vi "Get Plot at Mouse Click in Plot Area [AAC].vi"(8 "error in (no error)":errorcluster, 10 "Mouse Click Coordinates (defaut: last plot)":T2={"Horizontal"=2147483647, "Vertical"=0}, 11 "XYGraph Ref":T1) -> (0 "error out":errorcluster, 1 "Plot Index":i32, 3 "XYGraph Ref":T1)   [LabVIEW 2019]
doc: "If the Mouse Coordinates X value = 2147483647 (max I32 value), this means that the last plot is sought for is thus the plot returned.\nIf there is no plot in the Graph, -1 is returned"
uses:
  XY Graph/XY Graph Refnum.ctl
  <vilib>/Utility/miscctls.llb/LVPoint32TypeDef.ctl
  XY Graph/XY Graph Add-Ons.lvlib
panel:
  in  "Array of Array Cluster":cluster{"Array":dbl[], "Array":dbl[]}[](array[cluster])
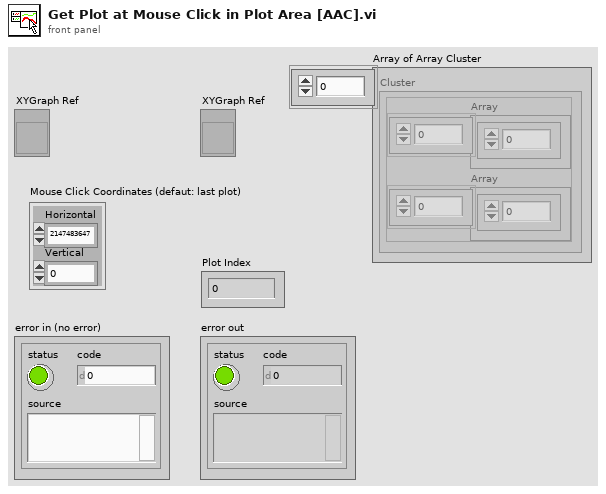
[diagram p1: front panel]
types:
  T1 = typedef "XY Graph Add-Ons.lvlib/XY Graph Refnum.ctl" = refnum<vi>
  T2 = typedef "LVPoint32TypeDef.ctl" = cluster{"Horizontal":i32, "Vertical":i32}
  T3 = typedef "LVRectTypeDef.ctl" = cluster{"Left":i16, "Top":i16, "Right":i16, "Bottom":i16}
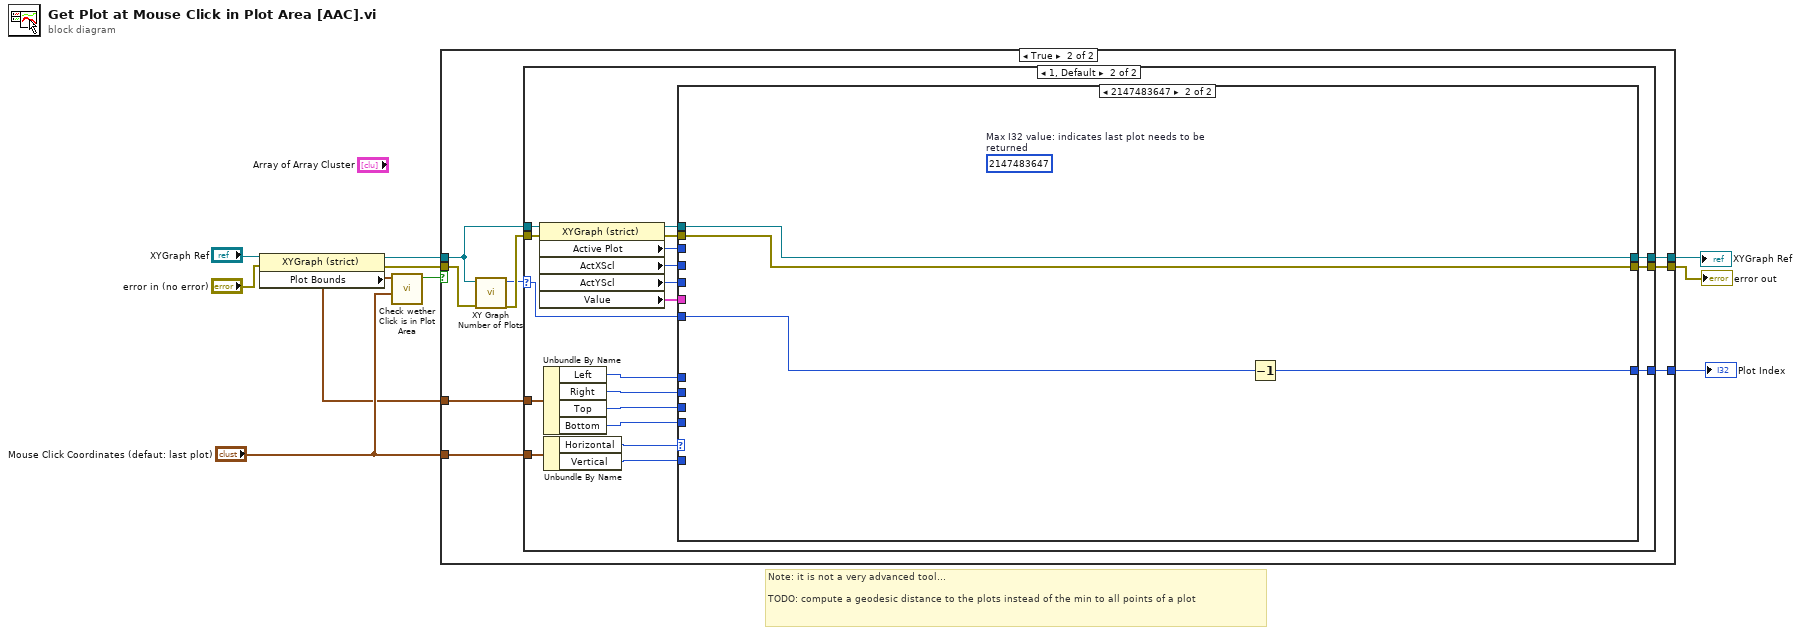
[diagram p0: block diagram]
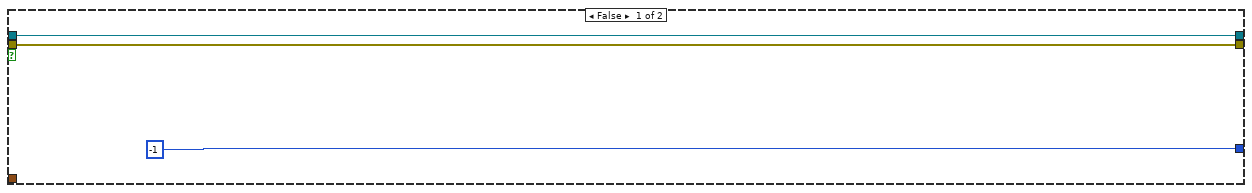
[diagram p2: hidden frame]
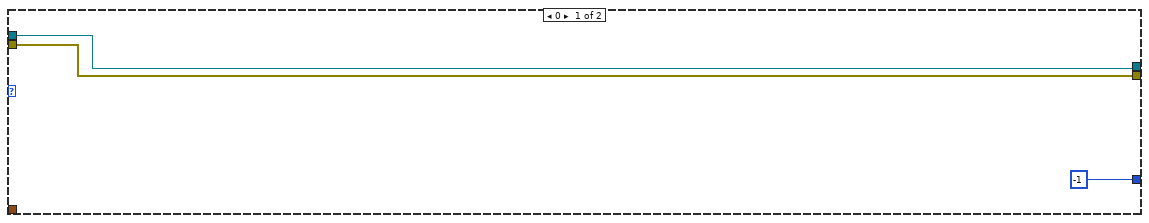
[diagram p3: hidden frame]
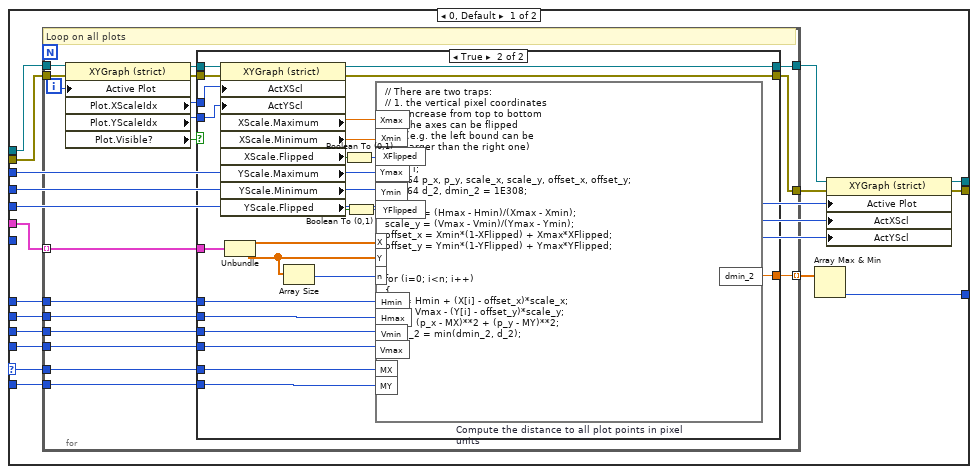
[diagram p4: hidden frame]
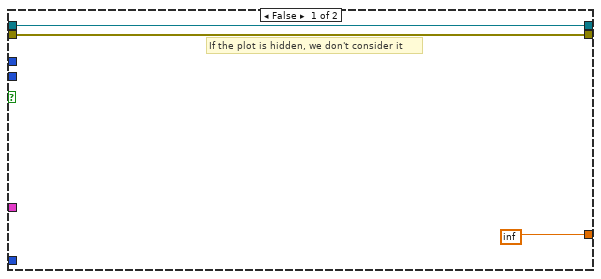
[diagram p5: hidden frame]
diagram:
  # "Note: it is not a very advanced tool...\n\nTODO: compute a geodesic distance to the plots instead of the min to all points of a plot"
  n1 = property class="XYGraph (strict)"(reference="XYGraph Ref", error in="error in (no error)") -> (reference out=w6:T1, error out=w7:errorcluster, "Plot Bounds"=w1:T3)
  n2 = call "Check wether Click is in Plot Area.vi"("Mouse Click Coordinates"="Mouse Click Coordinates (defaut: last plot)", "Plot Bounds"=w1) -> ("Is in Plot Area?"=w8:bool)  [unwired: 9 in]
  n3 = case shown="True" w8 {
    tunnel: w7 -> [w12 w16]
    tunnel: w6 -> [w13 w17]
    tunnel: [w13 w22] -> w5
    tunnel: [w12 w21] -> w4
    tunnel: [-1 ("Plot Index") w18] -> w3
    tunnel: "Mouse Click Coordinates (defaut: last plot)" -> [_ w20]
    tunnel: w1 -> [_ w19]
    frame False {
    }
    frame True {
      n4 = call "XY Graph Number of Plots.vi"("Error In"=w16, "XYGraph in"=w17) -> ("Error Out"=w15:errorcluster, "# Plots"=w14:i32)  [unwired: 8 in]
      n5 = case shown="1, Default" w14 {
        selector: w14 -> [_ w26]
        tunnel: [w24 w45] -> w22
        tunnel: [w23 w44] -> w21
        tunnel: w20 -> [_ w43]
        tunnel: w19 -> [_ w42]
        tunnel: [-1 w41] -> w18
        tunnel: w17 -> [w24 w29]
        tunnel: w15 -> [w23 w28]
        frame 0 {
        }
        frame 1, Default {
          n6 = property class="XYGraph (strict)"(reference=w29, error in=w28) -> (reference out=w40:T1, error out=w27:errorcluster, "Active Plot"=w39:u32, "ActXScl"=w38:i32, "ActYScl"=w37:i32, "Value"=w30:cluster{"X Array":dbl[], "Y Array":dbl[]}[])
          n7 = Unbundle By Name(w42) -> ("Left"=w36:i16, "Right"=w35:i16, "Top"=w34:i16, "Bottom"=w33:i16)
          n8 = Unbundle By Name(w43) -> ("Horizontal"=w32:i32, "Vertical"=w31:i32)
          n9 = case shown="2147483647" w32 {
            selector: w32 -> [w52 _]
            tunnel: [w63 w111] -> w45
            tunnel: [w62 w110] -> w44
            tunnel: [w61 w112] -> w41
            tunnel: w40 -> [w60 w111]
            tunnel: w39 -> [w59 _]
            tunnel: w38 -> [w58 _]
            tunnel: w37 -> [w57 _]
            tunnel: w36 -> [w56 _]
            tunnel: w35 -> [w55 _]
            tunnel: w34 -> [w54 _]
            tunnel: w33 -> [w53 _]
            tunnel: w31 -> [w51 _]
            tunnel: w30 -> [w50 _]
            tunnel: w27 -> [w47 w110]
            tunnel: w26 -> [_ w113]
            frame 0, Default {
              n10 = for {
                tunnel: w50 -> [w81] mode=indexing
                tunnel: w60 -> [w68]
                tunnel: [w76] -> w49
                tunnel: w56 -> [w75]
                tunnel: w55 -> [w74]
                tunnel: w54 -> [w73]
                tunnel: w53 -> [w72]
                tunnel: w52 -> [w71]
                tunnel: w51 -> [w70]
                tunnel: [w69] -> w48 mode=indexing
                tunnel: w47 -> [w66]
                tunnel: [w64] -> w46
                i -> [w80]
                # "Loop on all plots"
                n11 = property class="XYGraph (strict)"(reference=w68, error in=w66, "Active Plot"=w80) -> (reference out=w79:T1, error out=w65:errorcluster, "Plot.XScaleIdx"=w78:u32, "Plot.YScaleIdx"=w77:u32, "Plot.Visible?"=w67:bool)
                n12 = case shown="True" w67 {
                  tunnel: w81 -> [_ w109]
                  tunnel: w79 -> [w84 w108]
                  tunnel: w78 -> [_ w107]
                  tunnel: w77 -> [_ w106]
                  tunnel: [w84 w105] -> w76
                  tunnel: w75 -> [_ w100]
                  tunnel: w74 -> [_ w99]
                  tunnel: w73 -> [_ w98]
                  tunnel: w72 -> [_ w97]
                  tunnel: w71 -> [_ w96]
                  tunnel: w70 -> [_ w95]
                  tunnel: [inf w93] -> w69
                  tunnel: w65 -> [w82 w86]
                  tunnel: [w82 w85] -> w64
                  frame False {
                    # "If the plot is hidden, we don't consider it"
                  }
                  frame True {
                    n13 = property class="XYGraph (strict)"(reference=w108, error in=w86, "ActXScl"=w107, "ActYScl"=w106) -> (reference out=w105:T1, error out=w85:errorcluster, "XScale.Maximum"=w104:dbl, "XScale.Minimum"=w103:dbl, "XScale.Flipped"=w92:bool, "YScale.Maximum"=w102:dbl, "YScale.Minimum"=w101:dbl, "YScale.Flipped"=w90:bool)
                    n14 = Unbundle(w109) -> ("X Array"=w94:dbl[], "Y Array"=w88:dbl[])
                    n15 = Array Size(array=w88) -> (size(s)=w87:i32)
                    n16 = Boolean To (0,1)(Boolean=w92) -> (0, 1=w91:i16)
                    n17 = Boolean To (0,1)(Boolean=w90) -> (0, 1=w89:i16)
                    n18 = formula code="// There are two traps:\n// 1. the vertical pixel coordinates\n//     increase from top to bottom\n// 2. the axes can be flipped\n//     (e.g. the left bound can be\n//     larger than the right one)\n\nint32 i;\nfloat64 p_x, p_y, scale_x, scale_y, offset_x, offset_y;\nfloat64 d_2, dmin_2 = 1E308;\n\nscale_x = (Hmax - Hmin)/(Xmax - Xmin);\nscale_y = (Vmax - Vmin)/(Ymax - Ymin);\noffset_x = Xmin*(1-XFlipped) + Xmax*XFlipped;\noffset_y = Ymin*(1-YFlipped) + Ymax*YFlipped;\n\n\nfor (i=0; i<n; i++)\n{\np_x = Hmin + (X[i] - offset_x)*scale_x;\np_y = Vmax - (Y[i] - offset_y)*scale_y;\nd_2 = (p_x - MX)**2 + (p_y - MY)**2;\ndmin_2 = min(dmin_2, d_2);\n}" "Compute the distance to all plot points in pixel units"("Xmax"=w104, "Xmin"=w103, "Ymax"=w102, "Ymin"=w101, "Hmin"=w100, "Hmax"=w99, "Vmin"=w98, "Vmax"=w97, "MX"=w96, "MY"=w95, "X"=w94, "Y"=w88, "XFlipped"=w91, "YFlipped"=w89, "n"=w87) -> ("dmin_2"=w93:dbl)
                  }
                }
              }
              n19 = Array Max & Min(array=w48) -> (min index (indices)=w61:i32)  [unwired: 3 out]
              n20 = property class="XYGraph (strict)"(reference=w49, error in=w46, "Active Plot"=w59, "ActXScl"=w58, "ActYScl"=w57) -> (reference out=w63:T1, error out=w62:errorcluster)
            }
            frame 2147483647 {
              (unwired) 2147483647  # Max I32 value: indicates last plot needs to be returned
              n21 = Decrement(x=w113) -> (x-1=w112:i32)
            }
          }
        }
      }
    }
  }
  "Plot Index" <- w3
  "XYGraph Ref" <- w5
  "error out" <- w4
